vi "Init Block.vi"(8 "Worker VI":refnum<vi>) -> (0 "error out":errorcluster, 1 "Command Queue":refnum<queue>, 2 "Depth":i32, 3 "Status Queue":refnum<queue>)   [LabVIEW 2020, in "FlexBlocks.lvlib"]
uses:
  FlexBlocks.lvlib
  Command.ctl
  Block Status with Error.ctl
  Block Status.ctl
  Block State.ctl
  Run Action.ctl
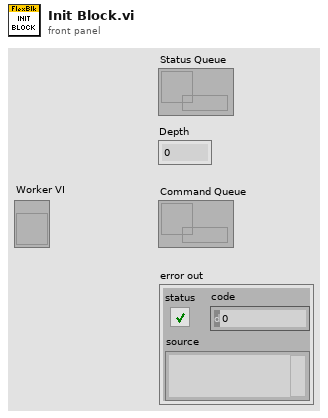
[diagram p1: front panel]
types:
  T1 = typedef "FlexBlocks.lvlib/Block Status with Error.ctl" = cluster{"Status":T2, "Error":errorcluster}
  T2 = typedef "FlexBlocks.lvlib/Block Status.ctl" = cluster{"State":T3, "i":i32, "Init":bool, "Started":bool, "Action":T4}
  T3 = typedef "FlexBlocks.lvlib/Block State.ctl" = enum16{"Idle", "Init", "Start", "Run", "Stop"}
  T4 = typedef "FlexBlocks.lvlib/Run Action.ctl" = enum16{"N/A", "Read", "Work", "Write"}
  T5 = typedef "FlexBlocks.lvlib/Command.ctl" = enum16{"Close", "Step", "Run", "Pause", "Init"}
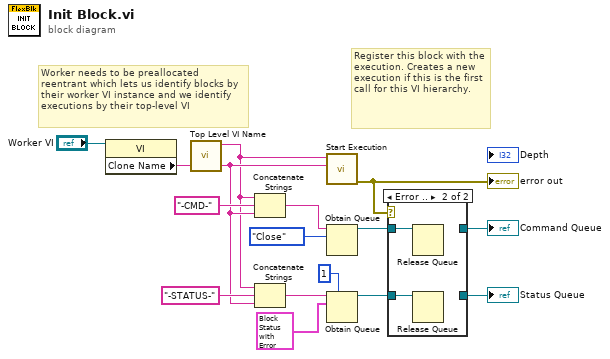
[diagram p0: block diagram]
diagram:
  # "Worker needs to be preallocated reentrant which lets us identify blocks by their worker VI instance and we identify executions by their top-level VI"
  # "Register this block with the execution. Creates a new execution if this is the first call for this VI hierarchy."
  n1 = property class="VI"(reference="Worker VI") -> ("Clone Name"=w3:string)  [unwired: 1 in, 2 out]
  n2 = call "Top Level VI Name.vi"() -> ("Top Level VI Name"=w1:string)  [unwired: 11 in]
  n3 = Concatenate Strings(w1, "-CMD-" ("string"), w3) -> (w15:string)
  n4 = Concatenate Strings(w1, "-STATUS-" ("string"), w3) -> (w12:string)
  n5 = call "Start Execution.vi"("Block Instance"=w3, "Hierarchy"=w1) -> ("error out"=w2:errorcluster)  [unwired: 9 in]
  "error out" <- w2
  n6 = Obtain Queue(name (unnamed)=w15, element data type=Command."Close" ("Command")) -> (queue out=w5:refnum<queue>)  [unwired: 3 in, 2 out]
  n7 = Obtain Queue(max queue size (-1, unlimited)=1, name (unnamed)=w12, element data type=T1 {"Status"={"State"=enum."Init", "i"=0, "Init"=FALSE, "Started"=FALSE, "Action"=enum."N/A"}, "Error"={"status"=FALSE, "code"=0, "source"=""}} ("Block Status with Error")) -> (queue out=w4:refnum<queue>)  [unwired: 2 in, 2 out]
  n8 = case shown="Error .." w2 {
    tunnel: [w17 _] -> w13
    tunnel: w5 -> [w17 w19]
    tunnel: [w16 _] -> w7
    tunnel: w4 -> [w16 w18]
    frame No Error {
    }
    frame Error {
      n9 = Release Queue(queue=w19) -> ()  [unwired: 2 in, 3 out]
      n10 = Release Queue(queue=w18) -> ()  [unwired: 2 in, 3 out]
    }
  }
  "Command Queue" <- w13
  "Status Queue" <- w7
